vi "2_Waveform_Signal_Classifier(Inference).vi"() -> ()   [LabVIEW 2020]
uses:
  <vilib>/Ngene/DeepLTK/Toolkit/NN_Network/Controls/NN_Save_Before_Destroy_Options.ctl
  <vilib>/Ngene/DeepLTK/Toolkit/NN_Layers/Layers/Input/API/NN_Layer_Set_Out(Input1D_idx).vi
  <vilib>/Ngene/DeepLTK/Toolkit/Deep_Learning_Toolkit_by_Ngene.lvlib
  <vilib>/measure/NI_MABase.lvlib
panel:
  out "Labels":string[](array[string])=["Triangle Wave", "Square Wave", "Sine Wave", "Sawtooth Wave", "Noise"]
  in  "Offset":dbl=0.2 format="%0.2p"
  out "Generated WaveForm":waveform(dbl)(graph)={"t0"=timestamp(0 s since 1904-01-01), "dt"=0.001, "Y"=[1.2, 1.2, 1.2, 1.2, -0.8, -0.8, -0.8, -0.8, -0.8, -0.8, 1.2, 1.2, 1.2, 1.2, 1.2, 1.2, 1.2, -0.8, -0.8, -0.8, -0.8, -0.8, -0.8, 1.2, 1.2, 1.2, 1.2, 1.2, 1.2, -0.8, -0.8, -0.8, -0.8, -0.8, -0.8, -0.8, 1.2, 1.2, 1.2, 1.2, 1.2, 1.2, -0.8, -0.8, -0.8, -0.8, -0.8, -0.8, -0.8, 1.2, 1.2, 1.2, 1.2, 1.2, 1.2, -0.8, -0.8, -0.8, -0.8, -0.8, -0.8, 1.2, 1.2, 1.2, 1.2, 1.2, 1.2, 1.2, -0.8, -0.8, -0.8, -0.8, -0.8, -0.8, 1.2, 1.2, 1.2, 1.2, 1.2, 1.2, 1.2, -0.8, -0.8, -0.8, -0.8, -0.8, -0.8, 1.2, 1.2, 1.2, 1.2, 1.2, 1.2, -0.8, -0.8, -0.8, -0.8, -0.8, -0.8, -0.8]}
  in  "Phase":dbl=90.0 format="%.2p"
  in  "Signal Type":T1(ring)=enum."Square Wave"
  in  "Amplitude":dbl=1.0
  in  "Frequency":dbl=78.0
  in  "Weight File Path":path=path "D:/Ngene/Projects_SVN/DeepLTK/Examples/2_Waveform_Processing/21_Waveform_Signal_Classifier/working/WF_Classifier/WF_Classifier_weights_23_09_22__19_08_43.bin"
  in  "Network Configuration File Path":path=path "D:/Ngene/Projects_SVN/DeepLTK/Examples/2_Waveform_Processing/21_Waveform_Signal_Classifier/working/WF_Classifier/WF_Classifier_net_cfg_23_09_22__19_08_43.cfg"
  out "Class Probability":sgl[](array[slide])=[0.01863354, 0.98447204, 8.268769e-15, 9.205111e-07, 5.3137904e-14] scale=0.0..1.0
  in  "Stop":bool
  # "Overview: Demonstrates the usage of Deep Learning Toolkit for loading the model pretrained for waveform signal classification and running for inference.\nRequirements: DeepLTK - Deep Learning Toolkit for LabVIEW (https://www.ngene.co/deep-learning-toolkit-for-labview)\nInstructions:\n1. Provide Network Configuration File Path and Weight File Path generated from 1_Waveform_Signal_Classifier(Trainng).vi.\n2. Run the VI\n3. Input Waveform parameters and observe the prediction results.\n4. Press the Stop button to stop the VI.\n\nMore Examples:  https://github.com/ngenehub/deepltk_examples"
  # "Signal Generation"
  # "Predictions"
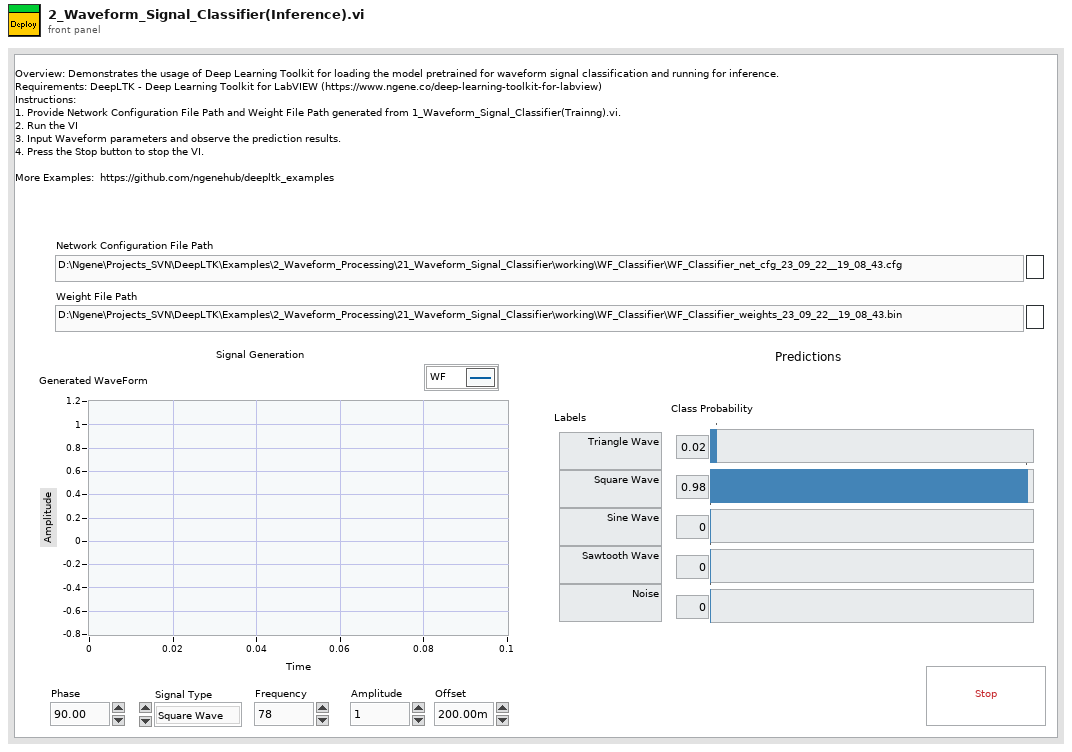
[diagram p1: front panel]
types:
  T1 = enum16{"Sine Wave", "Triangle Wave", "Square Wave", "Sawtooth Wave", "Noise"}
  T2 = typedef "Deep_Learning_Toolkit_by_Ngene.lvlib/NN_Save_Before_Destroy_Options.ctl" = cluster{"CFG?":bool, "Weights?":bool, "Render?":bool}
  T3 = typedef "Deep_Learning_Toolkit_by_Ngene.lvlib/NN_Config_Params.ctl" = cluster{"Name":string, "mBatch":i32, "NN_Train_Params":T4, "LR_Decay_Policy":T7, "Labels":string[], "Loss":T9}
  T4 = typedef "Deep_Learning_Toolkit_by_Ngene.lvlib/NN_Train_Params.ctl" = cluster{"Optimizer":T5, "Beta_1":sgl, "Beta_2":sgl, "Weight Decay(L1)":sgl, "Weight Decay(L2)":sgl, "Data_Sampling":T6}
  T5 = typedef "Deep_Learning_Toolkit_by_Ngene.lvlib/NN_Train_Optimizer.ctl" = enum16{"SGD", "Adam", "Adagrad", "Adadelta", "RMSProp", "Nesterov"}
  T6 = typedef "Deep_Learning_Toolkit_by_Ngene.lvlib/NN_Train_Data_Sampling.ctl" = enum16{"Random", "Sequential"}
  T7 = typedef "Deep_Learning_Toolkit_by_Ngene.lvlib/NN_LR_Policy_Cfg.ctl" = cluster{"Policy_Type":T8, "LR0":dbl, "k":sgl, "WarmUp_Policy":enum16{"Step", "Ramp"}, "WarmUp_Iter":i32, "WarmUp_Ratio":sgl}
  T8 = typedef "Deep_Learning_Toolkit_by_Ngene.lvlib/NN_LR_Policy_Type.ctl" = enum16{"Manual", "Step", "Exp", "1/t"}
  T9 = typedef "Deep_Learning_Toolkit_by_Ngene.lvlib/NN_Loss_Config_Params.ctl" = cluster{"Loss_Type":T10, "Loss_Conf_Params":variant}
  T10 = typedef "Deep_Learning_Toolkit_by_Ngene.lvlib/NN_Loss_Type.ctl" = enum16{"None", "MSE", "CrossEntropy", "YOLO_v2"}
  T11 = typedef "Deep_Learning_Toolkit_by_Ngene.lvlib/NN_Layer_Config_Params.ctl" = cluster{"Layer_Type":T12, "Layer_Conf_Params":variant}
  T12 = typedef "Deep_Learning_Toolkit_by_Ngene.lvlib/NN_Layer_Type.ctl" = enum16{"Input1D", "Input3D", "Conv2D", "Conv2D_Adv", "MaxPool", "AvgPool", "UpSample", "DropOut3D", "ShortCut", "Concat", "SoftMax3D", "FC", "DropOut", "Softmax", "Flatten", "YOLO_v2", "Unsupported"}
  T13 = typedef "Deep_Learning_Toolkit_by_Ngene.lvlib/NN.ctl" = cluster{"Name":string, "No of Layers":i32, "mBatch":i32, "Layers":T14[], "Dimty":T15, "Dims_In":T16, "Dims_Out":T16, "Working_Dir":path, "Train?":bool, "Train_Params":T4, "LR_Update_Policy":T7, "Session Data":T17, "Ground_truth":T18, "NNg_hdls":T20, "NN_Device":T21, "GPU Id":i32, "Labels":string[], "Receptive Field":T22[], "Loss_Type":T10, "Loss_Cfg_Prms":variant}
  T14 = typedef "Deep_Learning_Toolkit_by_Ngene.lvlib/NN_Layer_ref.ctl" = refnum<data-value>
  T15 = typedef "Deep_Learning_Toolkit_by_Ngene.lvlib/NN_In_Out_Dim-ty.ctl" = enum8{"In1D_Out1D", "In3D_Out1D", "In3D_Out3D", "In3D_OutBBox"}
  T16 = typedef "Deep_Learning_Toolkit_by_Ngene.lvlib/NN_Dims(C,H,W).ctl" = cluster{"C":i32, "H":i32, "W":i32}
  T17 = typedef "Deep_Learning_Toolkit_by_Ngene.lvlib/NN_Train_Session_Data.ctl" = cluster{"Epochs":sgl, "Tot_Iter":i32, "LR":sgl, "LR_iter":i32}
  T18 = typedef "Deep_Learning_Toolkit_by_Ngene.lvlib/NN_Ground_truth.ctl" = cluster{"Y":variant, "Y_idx":T19}
  T19 = typedef "Deep_Learning_Toolkit_by_Ngene.lvlib/NN_Data_ref(1D_I32).ctl" = refnum<data-value>
  T20 = typedef "Deep_Learning_Toolkit_by_Ngene.lvlib/nng_cuda_handles.ctl" = cluster{"cudnn":u64, "cublas":u64, "stream":u64, "curand":u64}
  T21 = typedef "Deep_Learning_Toolkit_by_Ngene.lvlib/NN_Device.ctl" = enum16{"CPU", "GPU"}
  T22 = typedef "Deep_Learning_Toolkit_by_Ngene.lvlib/NN_Dims(V,H).ctl" = cluster{"V":i32, "H":i32}
  T23 = typedef "Deep_Learning_Toolkit_by_Ngene.lvlib/NN_Layer.ctl" = cluster{"Name":string, "Layer_Data":variant, "Layer_Type":T12, "Dims_In":T16, "Layers_In":variant, "Dims_Out":T16, "Layers_Out":variant, "Metrics":T24, "GPU_Data":variant, "mBatch":i32, "NN_Device":T21, "NNg_hdls":T20, "Train?":bool, "Dimty":T25, "RecptField":T26}
  T24 = typedef "Deep_Learning_Toolkit_by_Ngene.lvlib/NN_Layer_Metrics.ctl" = cluster{"Data":dbl, "Params":dbl, "Ops":dbl}
  T25 = typedef "Deep_Learning_Toolkit_by_Ngene.lvlib/NN_Layer_Dimty.ctl" = enum16{"1D", "3D"}
  T26 = typedef "Deep_Learning_Toolkit_by_Ngene.lvlib/NN_Layer_RF_State.ctl" = cluster{"Dims":T22, "J":T22}
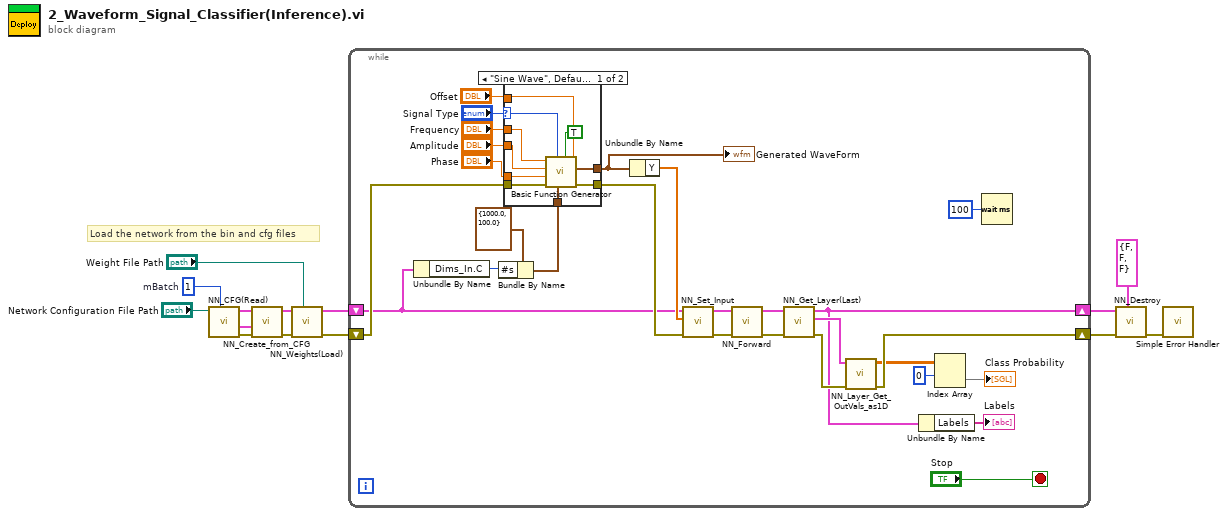
[diagram p0: block diagram]
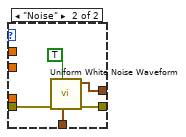
[diagram p2: hidden frame]
diagram:
  w1 = 1  # mBatch
  # "Load the network from the bin and cfg files"
  n1 = call <vilib>:"NN_CFG(Read).vi"("mBatch"=w1, "CFG file path"="Network Configuration File Path") -> ("error out"=w8:errorcluster, "Net_Cfg"=w9:T3, "Layer_Cfg"=w7:T11[])  [unwired: 7 in]
  n2 = call <vilib>:"NN_Create_from_CFG.vi"("error in (no error)"=w8, "Net_Cfg"=w9, "Layer_Cfg"=w7) -> ("error out"=w11:errorcluster, "NN out"=w6:T13)  [unwired: 7 in]
  n3 = call <vilib>:"NN_Weights(Load).vi"("Weight File Path"="Weight File Path", "error in (no error)"=w11, "NN in"=w6) -> ("error out"=w5:errorcluster, "NN out"=w4:T13)  [unwired: 7 in]
  n4 = while {
    shift-right: [w40] -> w14
    shift-left: w5 -> [w41]
    shift-right: [w18] -> w13
    shift-left: w4 -> [w21]
    stop <- "Stop" stop-if-true
    n5 = Unbundle By Name(w21) -> ("Dims_In.C"=w19:i32)
    n6 = Bundle By Name(cluster=cluster{"Fs":dbl, "#s":dbl} {"Fs"=1000.0, "#s"=100.0} ("sampling info"), "#s"=w19) -> (w20:cluster{"Fs":dbl, "#s":dbl})
    n7 = case shown="\"Sine Wave\", Default" "Signal Type" {
      selector: "Signal Type" -> [w46 _]
      tunnel: w41 -> [w51 w56]
      tunnel: "Frequency" -> [w50 _]
      tunnel: "Amplitude" -> [w49 _]
      tunnel: [w48 w53] -> w28
      tunnel: [w47 w54] -> w15
      tunnel: "Phase" -> [w45 _]
      tunnel: "Offset" -> [w44 _]
      tunnel: w20 -> [w42 w55]
      frame "Sine Wave", Default {
        n8 = call <vilib>:"Basic Function Generator.vi"("offset"=w44, "reset signal"=TRUE, "sampling info"=w42, "signal type"=w46, "error in (no error)"=w51, "phase"=w45, "amplitude"=w49, "frequency"=w50) -> ("error out"=w48:errorcluster, "signal out"=w47:waveform(dbl))  [unwired: 1 in, 1 out]
      }
      frame "Noise" {
        n9 = call <vilib>:"Uniform White Noise Waveform.vi"("sampling info"=w55, "reset signal"=TRUE, "error in (no error)"=w56) -> ("error out"=w53:errorcluster, "signal out"=w54:waveform(dbl))  [unwired: 7 in]
      }
    }
    "Generated WaveForm" <- w15
    n10 = Unbundle By Name(w15) -> ("Y"=w27:dbl[])
    n11 = call-poly <vilib>:"NN_Set_Input.vi"("error in (no error)"=w28, "Data_In(1D_SGL)"=w27, "NN In"=w21) -> ("error out"=w39:errorcluster, "NN Out"=w36:T13)  [unwired: 7 in]
    n12 = call <vilib>:"NN_Forward.vi"("error in (no error)"=w39, "NN in"=w36) -> ("error out"=w38:errorcluster, "NN out"=w37:T13)  [unwired: 6 in, 2 out]
    n13 = call <vilib>:"NN_Get_Layer(Last).vi"("error in (no error)"=w38, "NN in"=w37) -> ("error out"=w35:errorcluster, "Last_Layer"=w34:T23, "NN out"=w18:T13)  [unwired: 6 in, 1 out]
    n14 = call <vilib>:"NN_Layer_Get_OutVals_as1D.vi"("error in (no error)"=w35, "Layer"=w34) -> ("error out"=w40:errorcluster, "Out(as1D)"=w33:sgl[][])  [unwired: 8 in]
    n15 = Unbundle By Name(w18) -> ("Labels"=→"Labels":string[])
    n16 = Index Array(array=w33, index (row)=0) -> (element=→"Class Probability":sgl[])  [unwired: 1 in]
    n17 = Wait (ms)(milliseconds to wait=u32 100) -> ()  [unwired: 1 out]
  }
  n18 = call <vilib>:"NN_Destroy.vi"("Save (T, T, T)"=T2 {"CFG?"=FALSE, "Weights?"=FALSE, "Render?"=FALSE}, "error in (no error)"=w14, "NN in"=w13) -> ("error out"=w2:errorcluster)  [unwired: 8 in]
  n19 = call <vilib>:"Simple Error Handler.vi"("error in (no error)"=w2) -> ()  [unwired: 4 in, 5 out]
